vi "Control Paths.vi"(11 "VolatusControlsList in":refnum<class "VolatusControlsList.lvclass">) -> (2 "Control Paths":path[](array[path]))   [LabVIEW 2020, in "VolatusGUIEditorCore.lvlib" / "VolatusControlsList.lvclass"]
uses:
  VolatusControlsList.lvclass
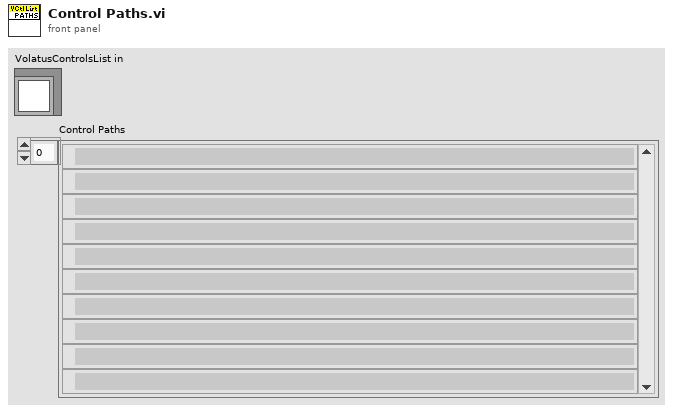
[diagram p1: front panel]
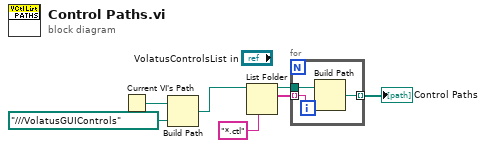
[diagram p0: block diagram]
diagram:
  n1 = Current VI's Path() -> (path=w3:path)
  n2 = Build Path(base path=w3, name or relative path=path "../../../VolatusGUIControls") -> (appended path=w1:path)
  n3 = List Folder(path=w1, pattern="*.ctl") -> (path out=w6:path, filenames=w5:string[])  [unwired: 2 in, 2 out]
  n4 = for {
    tunnel: w6 -> [w10]
    tunnel: w5 -> [w9] mode=indexing
    tunnel: [w8] -> w4 mode=indexing
    n5 = Build Path(base path=w10, name or relative path=w9) -> (appended path=w8:path)
  }
  "Control Paths" <- w4
